vi "Update Status.vi"(8 "error in (no error)":errorcluster, 10 "Team Status":T1, 11 "Team Dashboard Panel in":refnum<class "Team Dashboard Panel.lvclass">) -> (0 "error out":errorcluster, 3 "Team Dashboard Panel out":refnum<class "Team Dashboard Panel.lvclass">)   [LabVIEW 2020, in "SB App.lvlib" / "Team Dashboard Panel.lvclass"]
uses:
  Team Dashboard Panel.lvclass
  Team Status Data.ctl
  SquareBattle/Team Stats.ctl
  SquareBattle/Team State.ctl
  Team Dashboard Panel.lvclass/Team Dashboard Panel.ctl
  SquareBattle/SquareBattle.lvlib
  SB App.lvlib
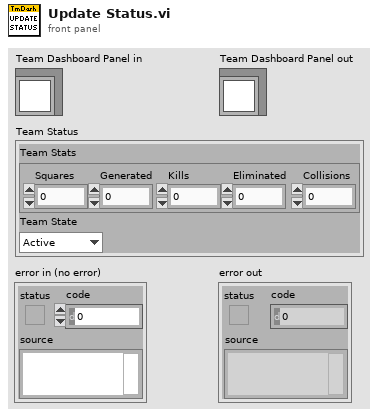
[diagram p1: front panel]
types:
  T1 = typedef "SB App.lvlib/Team Status Data.ctl" = cluster{"Team Stats":T2, "Team State":T3}
  T2 = typedef "SquareBattle.lvlib/Team Stats.ctl" = cluster{"Squares":i32, "Generated":i32, "Kills":i32, "Eliminated":i32, "Collisions":i32}
  T3 = typedef "SquareBattle.lvlib/Team State.ctl" = enum16{"Active", "Defeated", "Won"}
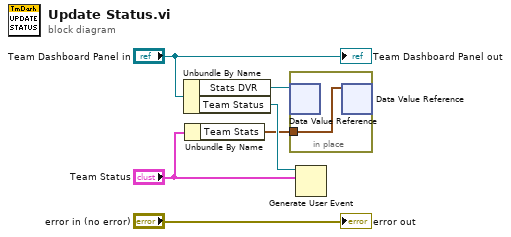
[diagram p0: block diagram]
diagram:
  n1 = Unbundle By Name("Team Dashboard Panel in") -> ("Stats DVR"=w3:refnum<data-value>, "Team Status"=w4:refnum<user-event>)
  n2 = Unbundle By Name("Team Status") -> ("Team Stats"=w1:T2)
  n3 = in-place {
    in-place-border: w1 -> [w7]
    n4 = in-place-dvr #1(w3) -> ()  [unwired: 2 out]
    n5 = in-place-dvr #1(w7) -> ()  [unwired: 2 out]
  }
  n6 = Generate User Event(user event=w4, event data cluster="Team Status") -> ()  [unwired: 2 in, 2 out]
  "error out" <- "error in (no error)"
  "Team Dashboard Panel out" <- "Team Dashboard Panel in"
